vi "GetGaitTiming.vi"(8 "error in (no error)":errorcluster, 11 "CAlexData2 in":refnum<class "CAlexData2.lvclass">) -> (0 "Stance/Swing":dbl, 1 "SwingTime":dbl, 2 "GaitTime":dbl, 3 "CAlexData2 out":refnum<class "CAlexData2.lvclass">, 5 "FileName":string)   [LabVIEW 2015, in "CAlexData2.lvclass"]
uses:
  CAlexData2.lvclass
  <vilib>/Analysis/baseanly.llb/Mean (DBL).vi
  ExpData/ExpData.lvclass
  <vilib>/Analysis/NI_AALBase.lvlib
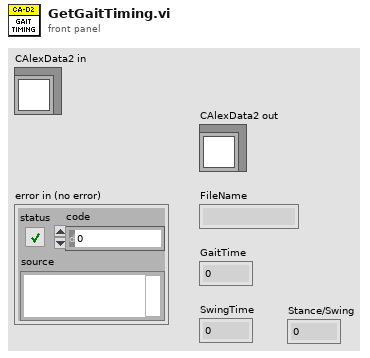
[diagram p1: front panel]
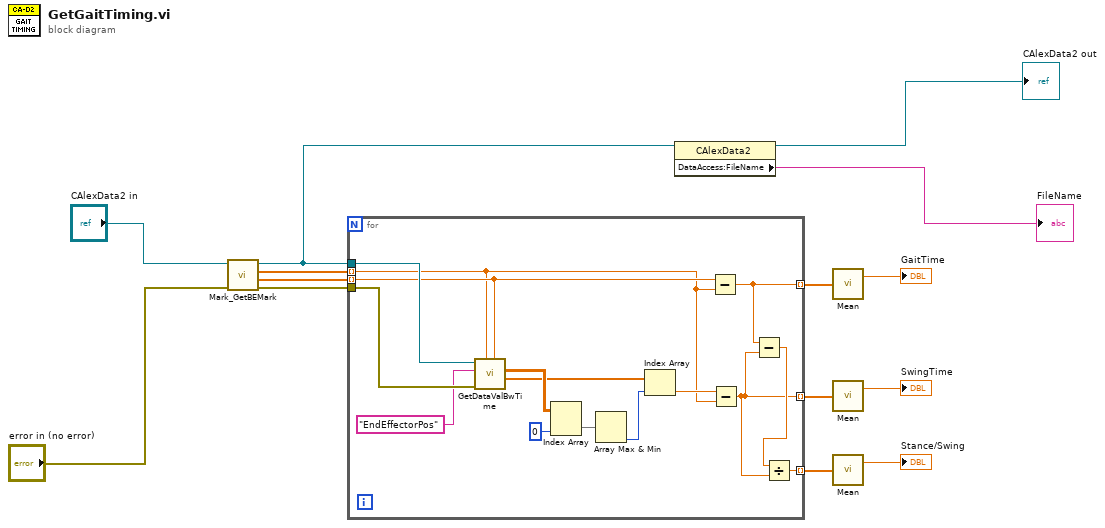
[diagram p0: block diagram]
diagram:
  n1 = call "Mark_GetBEMark.vi"("error in (no error)"="error in (no error)", "ExpData In"="CAlexData2 in") -> ("error out"=w5:errorcluster, "End"=w4:dbl[], "Begin"=w3:dbl[], "ExpData Out"=w9:refnum<class "CAlexData2.lvclass">)  [unwired: 5 in, 1 out]
  n2 = for {
    tunnel: w3 -> [w19] mode=indexing
    tunnel: w9 -> [w29]
    tunnel: w4 -> [w20] mode=indexing
    tunnel: w5 -> [w28]
    tunnel: [w17] -> w6 mode=indexing
    tunnel: [w15] -> w7 mode=indexing
    tunnel: [w18] -> w8 mode=indexing
    n3 = call-dynamic "GetDataValBwTime.vi"("Time End"=w20, "Time Begin"=w19, "error in (no error)"=w28, "Name"="EndEffectorPos", "ExpData in"=w29) -> ("Time Inbetween"=w23:dbl[], "Data Inbetween"=w26:dbl[][])  [unwired: 2 in, 3 out]
    n4 = Index Array(array=w26, index (col)=0 ("disabled index (col)")) -> (element=w24:dbl[])  [unwired: 1 in]
    n5 = Array Max & Min(array=w24) -> (min index (indices)=w22:i32)  [unwired: 3 out]
    n6 = Index Array(array=w23, index=w22) -> (element=w21:dbl)
    n7 = Subtract(x=w20, y=w19) -> (x-y=w17:dbl)
    n8 = Subtract(x=w21, y=w19) -> (x-y=w15:dbl)
    n9 = Subtract(x=w17, y=w15) -> (x-y=w16:dbl)
    n10 = Divide(x=w16, y=w15) -> (x/y=w18:dbl)
  }
  n11 = property class="CAlexData2"(reference=w9) -> (reference out=→"CAlexData2 out":refnum<class "CAlexData2.lvclass">, "DataAccess:FileName"=→"FileName":string)  [unwired: 1 in, 1 out]
  n12 = call-poly <vilib>:"Mean.vi"("X"=w6) -> ("mean"=→"GaitTime":dbl)  [unwired: 1 out]
  n13 = call-poly <vilib>:"Mean.vi"("X"=w7) -> ("mean"=→"SwingTime":dbl)  [unwired: 1 out]
  n14 = call-poly <vilib>:"Mean.vi"("X"=w8) -> ("mean"=→"Stance/Swing":dbl)  [unwired: 1 out]
